vi "PI Construct Limit String.vi"(11 "Limits":T1={"Limits On"=TRUE, "Limits"=[]}) -> (3 "Limit String":string)   [LabVIEW 2011]
uses:
  TypeDefs/PI Limit Parameters.ctl
  TypeDefs/PI Limit Definition.ctl
  TypeDefs/PI Limit Comparison.ctl
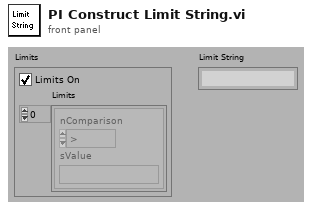
[diagram p1: front panel]
types:
  T1 = typedef "PI Limit Parameters.ctl" = cluster{"Limits On":bool, "Limits":T2[]}
  T2 = typedef "PI Limit Definition.ctl" = cluster{"nComparison":T3, "sValue":string}
  T3 = typedef "PI Limit Comparison.ctl" = enum16{">", ">=", "<", "<=", "<>", "="}
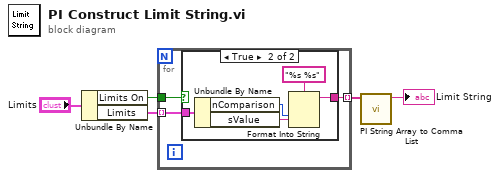
[diagram p0: block diagram]
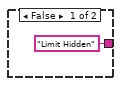
[diagram p2: hidden frame]
diagram:
  n1 = Unbundle By Name("Limits") -> ("Limits On"=w1:bool, "Limits"=w2:T2[])
  n2 = for {
    tunnel: w2 -> [w8] mode=indexing
    tunnel: [w7] -> w4 mode=indexing
    tunnel: w1 -> [w6]
    n3 = case shown="True" w6 {
      tunnel: w8 -> [_ w14]
      tunnel: ["Limit Hidden" ("format string") w10] -> w7
      frame False {
      }
      frame True {
        n4 = Unbundle By Name(w14) -> ("nComparison"=w12:T3, "sValue"=w11:string)
        n5 = Format Into String(format string="%s %s", w12, w11) -> (resulting string=w10:string)  [unwired: 2 in, 1 out]
      }
    }
  }
  n6 = call "PI String Array to Comma List.vi"("Array"=w4) -> ("String"=→"Limit String":string)  [unwired: 1 in, 9 out]
